vi "sub_play_DMD_mov_ext_trig.vi"(2 "Exposure (ms)":i32=1000, 3 "SequenceRepeats":i32=1, 4 "binary mov path":path=path "C:/Users/cohen_lab/Desktop/Labview_code/DMD_control/DMD6images.bin") -> ()   [LabVIEW 2012]
uses:
  C:/Program Files/ALP-4.1/ALP-4.1 high-speed API/Samples/alpD41.dll
panel:
  out "Dev Control Error":errorcluster
  out "Labview":errorcluster
  out "SeqControl3":errorcluster
  out "PicNum":i32
  out "DevFreeErr":i32
  out "SeqFreeErr":i32
  out "ProjWaitErr":i32
  out "ProjStartErr":i32
  out "SeqPutErr":i32
  out "SeqControl1":errorcluster
  out "SeqControl2":errorcluster
  out "SeqTimeErr":i32
  out "ProjControl":errorcluster
  out "SeqAllocErr":i32
  out "DevInq2":errorcluster
  out "DevInq1":errorcluster
  out "DevAllocErr":i32
  in  "Ext. Trig.":bool
  out "DMD Type":string
  out "SequID":u32
  out "DeviceID":u32
  out "SerialNumber":i32
  # "Initialization"
  # "Internal"
  # "External"
  # "0 = no error"
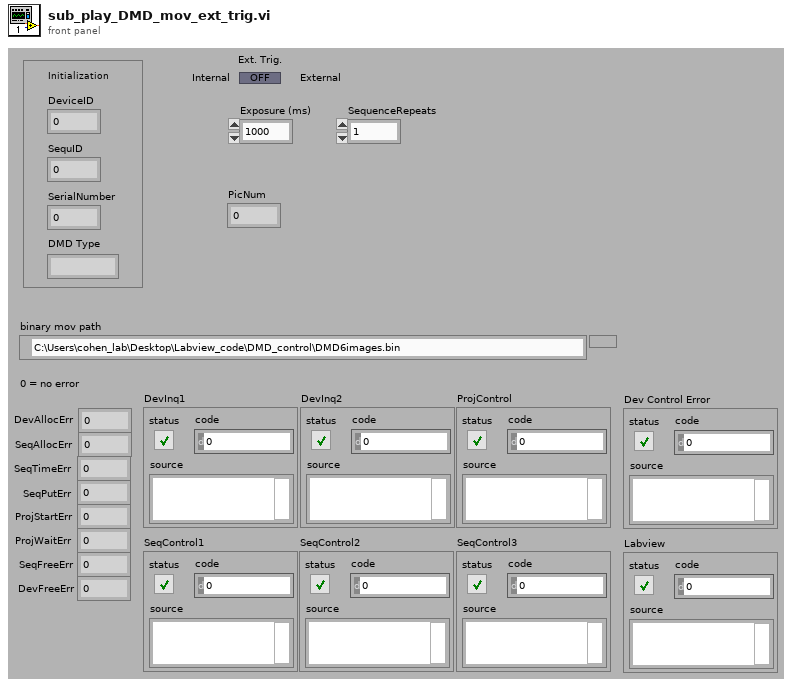
[diagram p1: front panel]
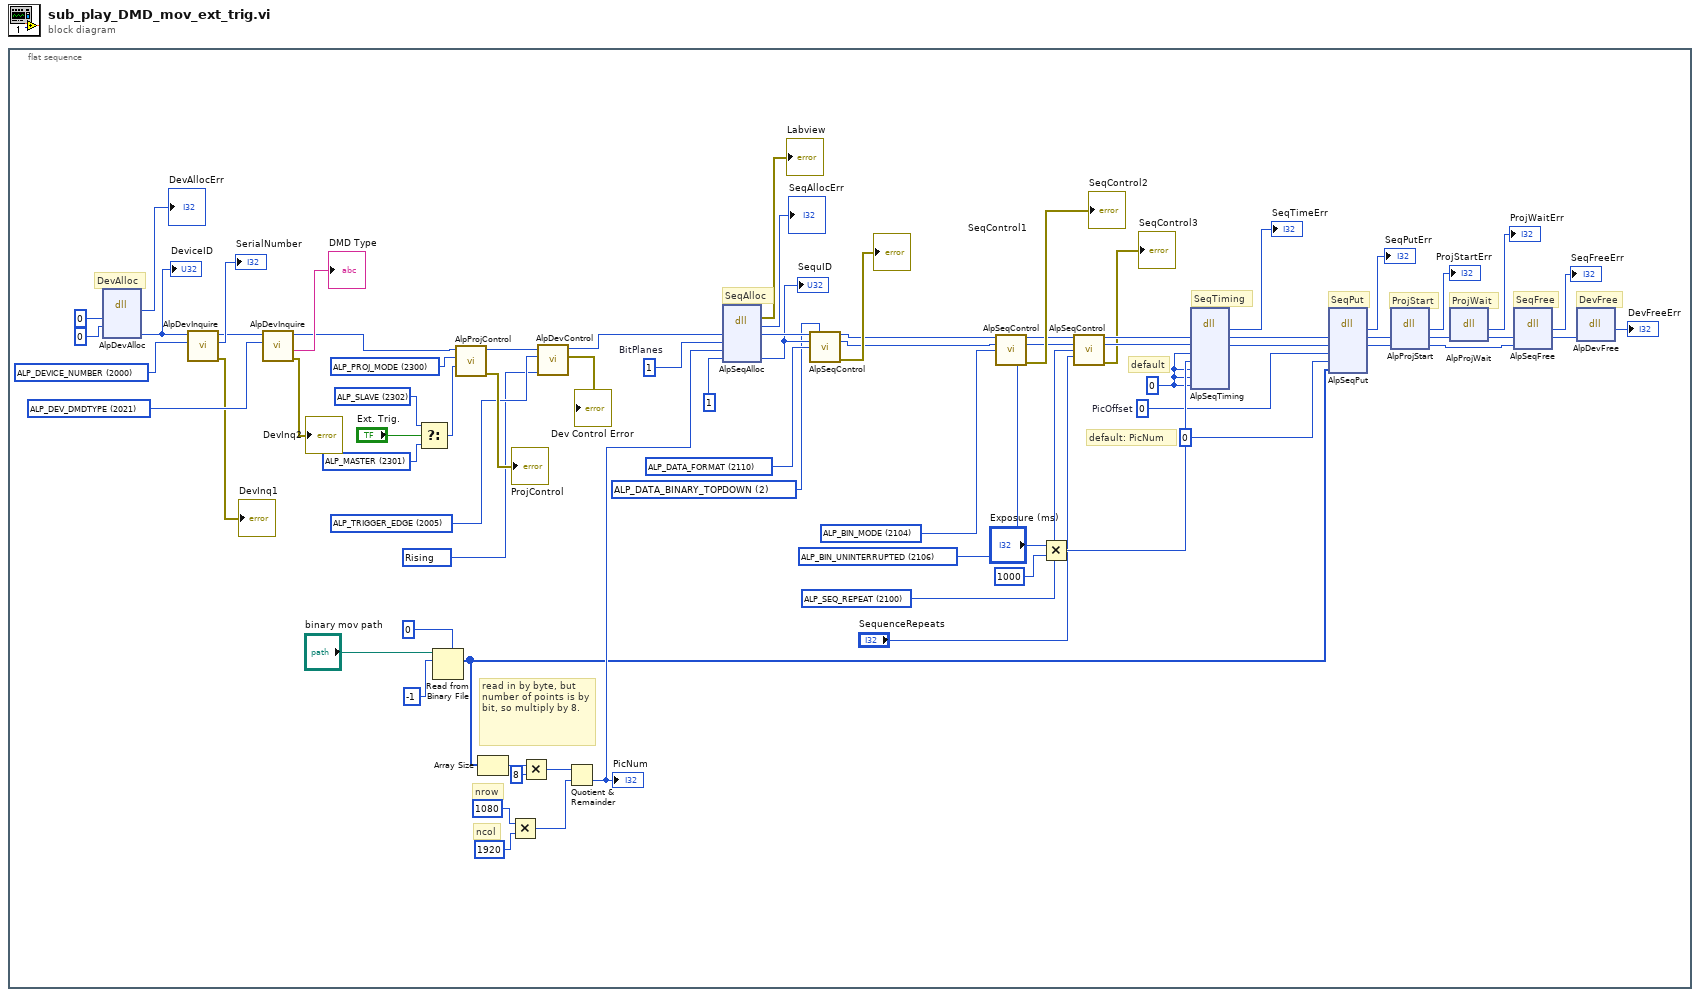
[diagram p0: block diagram]
diagram:
  n1 = flat-sequence {
    frame #0 {
      w3 = 2009 items=["Rising"=2009, "Falling"=2008] ("Trigger_Edge")
      w4 = 2005 items=["ALP_DEVICE_NUMBER"=2000, "ALP_VERSION"=2001, "ALP_DEV_STATE"=2002, "ALP_AVAIL_MEMORY"=2003, "ALP_SYNCH_POLARITY"=2004, "ALP_TRIGGER_EDGE"=2005, "ALP_USB_CONNECTION"=2016, "ALP_DEV_DMDTYPE"=2021, "ALP_DEV_DISPLAY_HEIGHT"=2057, "ALP_DEV_DISPLAY_WIDTH"=2058, "ALP_PWM_LEVEL"=2063, "ALP_DEV_DMD_MODE"=2064] ("InquireType")
      w14 = 2100 items=["ALP_SEQ_REPEAT"=2100, "ALP_FIRSTFRAME"=2101, "ALP_LASTFRAME"=2102, "ALP_BITNUM"=2103, "ALP_BIN_MODE"=2104, "ALP_DATA_FORMAT"=2110, "ALP_SEQ_PUT_LOCK"=2119] ("ControlType")
      w38 = 2300 items=["ALP_PROJ_MODE"=2300, "ALP_PROJ_INVERSION"=2306, "ALP_PROJ_UPSIDE_DOWN"=2307] ("ControlType")
      w21 = 2301 items=["ALP_MASTER"=2301, "ALP_SLAVE"=2302] ("ProjectorMode")
      w36 = 2302 items=["ALP_MASTER"=2301, "ALP_SLAVE"=2302] ("ProjectorMode")
      w46 = 2106 items=["ALP_BIN_NORMAL"=2105, "ALP_BIN_UNINTERRUPTED"=2106] ("Binary Mode")
      w47 = 2104 items=["ALP_SEQ_REPEAT"=2100, "ALP_FIRSTFRAME"=2101, "ALP_LASTFRAME"=2102, "ALP_BITNUM"=2103, "ALP_BIN_MODE"=2104, "ALP_DATA_FORMAT"=2110, "ALP_SEQ_PUT_LOCK"=2119] ("ControlType")
      w48 = 2 items=["ALP_DATA_MSB_ALIGN", "ALP_DATA_LSB_ALIGN", "ALP_DATA_BINARY_TOPDOWN", "ALP_DATA_BINARY_BOTTOMUP"] ("Data Format")
      w49 = 2110 items=["ALP_SEQ_REPEAT"=2100, "ALP_FIRSTFRAME"=2101, "ALP_LASTFRAME"=2102, "ALP_BITNUM"=2103, "ALP_BIN_MODE"=2104, "ALP_DATA_FORMAT"=2110, "ALP_SEQ_PUT_LOCK"=2119] ("ControlType")
      w55 = 0  # PicOffset
      w56 = 0
      w67 = 2021 items=["ALP_DEVICE_NUMBER"=2000, "ALP_VERSION"=2001, "ALP_DEV_STATE"=2002, "ALP_AVAIL_MEMORY"=2003, "ALP_SYNCH_POLARITY"=2004, "ALP_TRIGGER_EDGE"=2005, "ALP_USB_CONNECTION"=2016, "ALP_DEV_DMDTYPE"=2021, "ALP_DEV_DISPLAY_HEIGHT"=2057, "ALP_DEV_DISPLAY_WIDTH"=2058, "ALP_PWM_LEVEL"=2063, "ALP_DEV_DMD_MODE"=2064] ("InquireType")
      w69 = 2000 items=["ALP_DEVICE_NUMBER"=2000, "ALP_VERSION"=2001, "ALP_DEV_STATE"=2002, "ALP_AVAIL_MEMORY"=2003, "ALP_SYNCH_POLARITY"=2004, "ALP_TRIGGER_EDGE"=2005, "ALP_USB_CONNECTION"=2016, "ALP_DEV_DMDTYPE"=2021, "ALP_DEV_DISPLAY_HEIGHT"=2057, "ALP_DEV_DISPLAY_WIDTH"=2058, "ALP_PWM_LEVEL"=2063, "ALP_DEV_DMD_MODE"=2064] ("InquireType")
      w75 = 1  # BitPlanes
      # "read in by byte, but number of points is by bit, so multiply by 8."
      # "nrow"
      # "ncol"
      # "default: PicNum"
      # "ProjStart"
      # "SeqPut"
      # "ProjWait"
      # "default"
      # "SeqTiming"
      # "DevFree"
      # "SeqFree"
      # "DevAlloc"
      # "SeqAlloc"
      n2 = dll-call lib="C:/Program Files/ALP-4.1/ALP-4.1 high-speed API/Samples/alpD41.dll" fn="AlpDevAlloc"("DeviceNum"=0, "InitFlag"=0) -> ("return type"=→"DevAllocErr":i32, "DeviceIdPtr"=w71:u32)  [unwired: 6 in, 2 out]
      "DeviceID" <- w71
      n3 = call "AlpDevInquire.vi"("InquireType"=w69, "DeviceID"=w71) -> ("Error OUT"=→"DevInq1":errorcluster, "Output Number"=→"SerialNumber":i32, "DeviceIDout"=w68:u32)  [unwired: 6 in, 1 out]
      n4 = call "AlpDevInquire.vi"("InquireType"=w67, "DeviceID"=w68) -> ("Error OUT"=→"DevInq2":errorcluster, "Output Text"=→"DMD Type":string, "DeviceIDout"=w8:u32)  [unwired: 6 in, 1 out]
      n5 = Select(t=w36, s="Ext. Trig.", f=w21) -> (s? t:f=w35:i32)
      n6 = Read from Binary File(5:u8 0, 10:-1 ("count (1)"), 11:"binary mov path") -> (2:w22:u8[])  [unwired: 3 in, 3 out]
      n7 = call "AlpProjControl.vi"("ProjectorMode"=w35, "ControlType"=w38, "DeviceID"=w8) -> ("Error OUT"=→"ProjControl":errorcluster, "DeviceIDout"=w7:u32)  [unwired: 7 in]
      n8 = Array Size(array=w22) -> (size(s)=w19:i32)
      n9 = Multiply(x=1080, y=1920) -> (x*y=w25:i32)
      n10 = Multiply(x=w19, y=8) -> (x*y=w17:i32)
      n11 = call "AlpDevControl.vi"("Trigger_Edge"=w3, "InquireType"=w4, "DeviceID"=w7) -> ("Error OUT"=→"Dev Control Error":errorcluster, "DeviceId"=w5:u32)  [unwired: 7 in]
      n12 = Quotient & Remainder(x=w17, y=w25) -> (floor(x/y)=w23:i32)  [unwired: 1 out]
      "PicNum" <- w23
      n13 = dll-call lib="C:/Program Files/ALP-4.1/ALP-4.1 high-speed API/Samples/alpD41.dll" fn="AlpSeqAlloc"("DeviceId"=w5, "BitPlanes"=w75, "PicNum"=w23, "SequenceIdPtr"=u32 1) -> (error out=→"Labview":errorcluster, "return type"=→"SeqAllocErr":i32, "DeviceId"=w51:u32, "SequenceIdPtr"=w50:u32)  [unwired: 5 in, 1 out]
      "SequID" <- w50
      n14 = call "AlpSeqControl.vi"("DeviceID"=w51, "Data Format"=w48, "SequenceID"=w50, "ControlType"=w49) -> ("DeviceIDout"=w2:u32, "SequenceIDout"=w1:u32, "Error OUT"=→"SeqControl1":errorcluster)  [unwired: 9 in]
      n15 = call "AlpSeqControl.vi"("DeviceID"=w2, "SequenceID"=w1, "ControlType"=w47, "Binary Mode"=w46) -> ("DeviceIDout"=w16:u32, "SequenceIDout"=w15:u32, "Error OUT"=→"SeqControl2":errorcluster)  [unwired: 9 in]
      n16 = Multiply(x="Exposure (ms)", y=1000) -> (x*y=w59:i32)
      n17 = call "AlpSeqControl.vi"("DeviceID"=w16, "SequenceID"=w15, "ControlType"=w14, "SequenceRepeats"="SequenceRepeats") -> ("DeviceIDout"=w12:u32, "SequenceIDout"=w11:u32, "Error OUT"=→"SeqControl3":errorcluster)  [unwired: 9 in]
      n18 = dll-call lib="C:/Program Files/ALP-4.1/ALP-4.1 high-speed API/Samples/alpD41.dll" fn="AlpSeqTiming"("DeviceId"=w12, "SequenceId"=w11, "IlluminateTime"=w56, "PictureTime"=w59, "TriggerDelay"=w56, "TriggerPulseWidth"=w56, "VdDelay"=w56) -> ("return type"=→"SeqTimeErr":i32, "DeviceId"=w43:u32, "SequenceId"=w40:u32)  [unwired: 8 in, 2 out]
      n19 = dll-call lib="C:/Program Files/ALP-4.1/ALP-4.1 high-speed API/Samples/alpD41.dll" fn="AlpSeqPut"("DeviceId"=w43, "SequenceId"=w40, "PicOffset"=w55, "PicLoad"=0, "UserArrayPtr"=w22) -> ("return type"=→"SeqPutErr":i32, "DeviceId"=w42:u32, "SequenceId"=w41:u32)  [unwired: 6 in, 2 out]
      n20 = dll-call lib="C:/Program Files/ALP-4.1/ALP-4.1 high-speed API/Samples/alpD41.dll" fn="AlpProjStart" ("alpD40.dll:AlpProjStartCont")("DeviceId"=w42, "SequenceId"=w41) -> ("return type"=→"ProjStartErr":i32, "DeviceId"=w53:u32, "SequenceId"=w52:u32)  [unwired: 3 in, 2 out]
      n21 = dll-call lib="C:/Program Files/ALP-4.1/ALP-4.1 high-speed API/Samples/alpD41.dll" fn="AlpProjWait" ("Knoten zum Aufruf externer Bibliotheken")("DeviceId"=w53) -> ("return type"=→"ProjWaitErr":i32, "DeviceId"=w54:u32)  [unwired: 3 in, 2 out]
      n22 = dll-call lib="C:/Program Files/ALP-4.1/ALP-4.1 high-speed API/Samples/alpD41.dll" fn="AlpSeqFree"("DeviceId"=w54, "SequenceId"=w52) -> ("return type"=→"SeqFreeErr":i32, "DeviceId"=w72:u32)  [unwired: 4 in, 2 out]
      n23 = dll-call lib="C:/Program Files/ALP-4.1/ALP-4.1 high-speed API/Samples/alpD41.dll" fn="AlpDevFree"("DeviceId"=w72) -> ("return type"=→"DevFreeErr":i32)  [unwired: 4 in, 2 out]
    }
  }
